vi "main-20200210.vi"   [LabVIEW 2019]
uses:
  main_sm-20220210.ctl
types:
  T1 = typedef "main_sm-20220210.ctl" = enum16{"init", "color_vision", "goto_ball-can", "goto_ball-pool", "goto_home"}
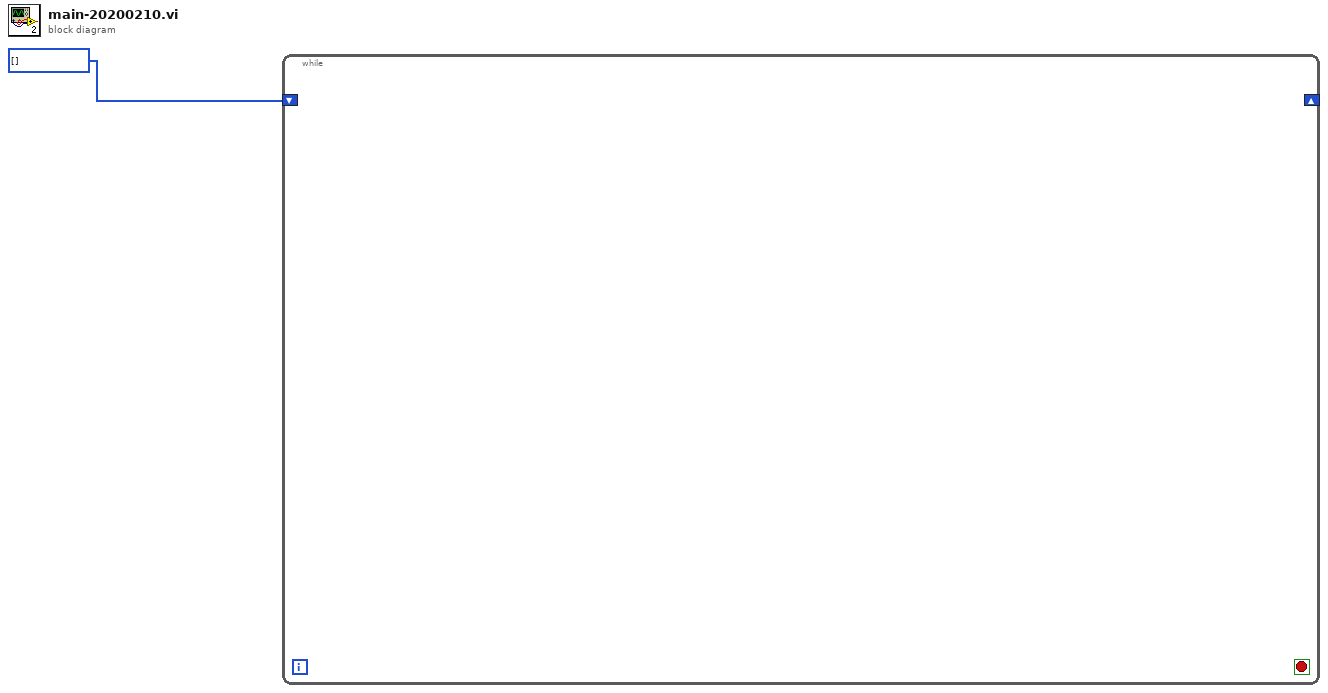
[diagram p0: block diagram]
diagram:
  w1 = T1[] [] items=["init", "color_vision", "goto_ball-can", "goto_ball-pool", "goto_home"]
  n1 = while {
    shift-right: _ -> [_]
    shift-left: w1 -> [_]
    stop <- _ stop-if-true
  }
